vi "Insert Into Array.vi"() -> ()   [LabVIEW 2014]
panel:
  out "输出二维数组":i32[][](array[numeric])
  out "输出一维数组":i32[](array[numeric])
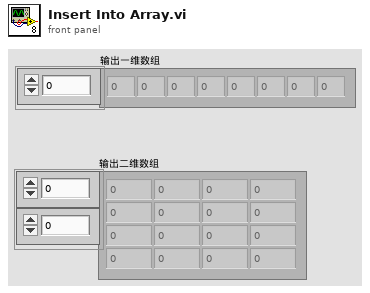
[diagram p1: front panel]
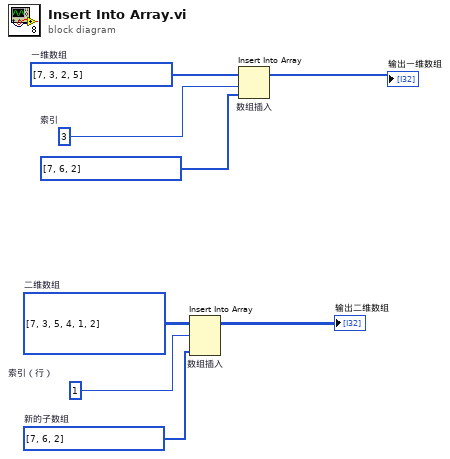
[diagram p0: block diagram]
diagram:
  w2 = i32[] [7, 6, 2]  # 新的子数组
  w4 = 1  # 索引（行）
  w7 = 3  # 索引
  w5 = i32[][] [[7, 3, 5], [4, 1, 2]]  # 二维数组
  w8 = i32[] [7, 3, 2, 5]  # 一维数组
  n1 = Insert Into Array "数组插入"(array=w5, index (row)=w4, new element=w2) -> (→"输出二维数组":i32[][])  [unwired: 1 in]
  n2 = Insert Into Array "数组插入"(array=w8, index=w7, new element=i32[] [7, 6, 2]) -> (→"输出一维数组":i32[])
